vi "beginDirectKickPlay.vi"(8 "error in (no error)":errorcluster, 10 "Game":refnum<class "Game.lvclass">, 11 "DirectKickPlay in":refnum<class "DirectKickPlay.lvclass">) -> (0 "error out":errorcluster, 2 "directKickBegin?":bool, 3 "DirectKickPlay out":refnum<class "DirectKickPlay.lvclass">)   [LabVIEW 2018, in "DirectKickPlay.lvclass"]
uses:
  DirectKickPlay.lvclass
  Game_class/Game.lvclass
  Utilities_class/Utilities.lvclass
  Referee_class/command_interpreted.ctl
  Team_class/OffensivePlay.ctl
  Game_class/Game.lvclass/Game.ctl
  Referee_class/Referee.lvclass/Referee.ctl
  Team_class/Team.lvclass/Team.ctl
  Game_class/Read OffensiveTeam.vi
  Team_class/Read OffensivePlay.vi
  Game_class/Read Referee.vi
  Referee_class/Read command_interpreted.vi
  Ally_class/Ally.lvclass
  Referee_class/Referee.lvclass
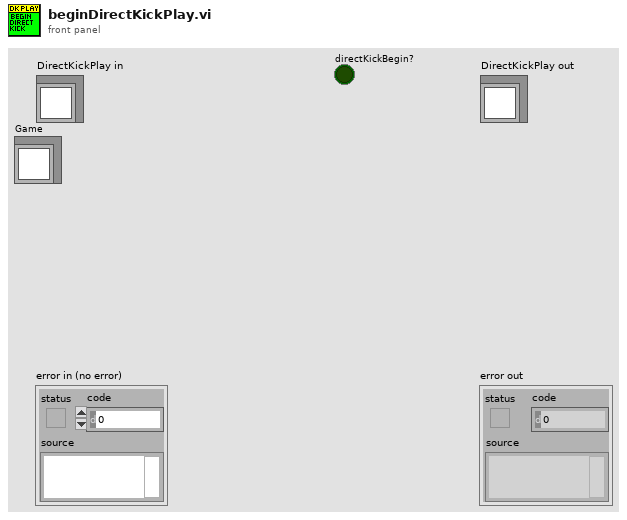
[diagram p1: front panel]
types:
  T1 = typedef "OffensivePlay.ctl" = enum16{"PreparePass", "PassToStriker", "BallOutOfField", "PassTo2ndStriker", "StopOffensive", "Prepare Penalty Enemy", "EnemyPossessionAtEnemyField", "EnemyPossesionAtOurField", "TestPlay", "PreparePenaltyAlly", "KickPenaltyAlly", "PrepareKickoffAlly", "PrepareKickoffEnemy", "IndirectEnemy", "DirectEnemy", "NormalGame", "DirectKick", "Pass", "Halt", "Timeout", "PassPlay", "PenaltyEnemy", "SimplePass"}
  T2 = typedef "command_interpreted.ctl" = enum16{"Goal Ally", "Goal Enemy", "Ball Placement Enemy", "Ball Placement Ally", "Normal Half Time", "Extra Time  Break", "Extra Half Time", "None", "Post Game", "PKA Normal Start", "Prepare Kickoff Ally", "PKE Normal Start", "Prepare Kickoff Enemy", "Force Start", "Halt", "Timeout", "Prepare Penalty Ally", "Prepare Penalty Enemy", "PPA NormalStart", "PPE Normal Start", "Indirect Free Ally", "Direct Free Enemy", "Direct Free Ally", "Indirect Free Enemy", "Stop"}
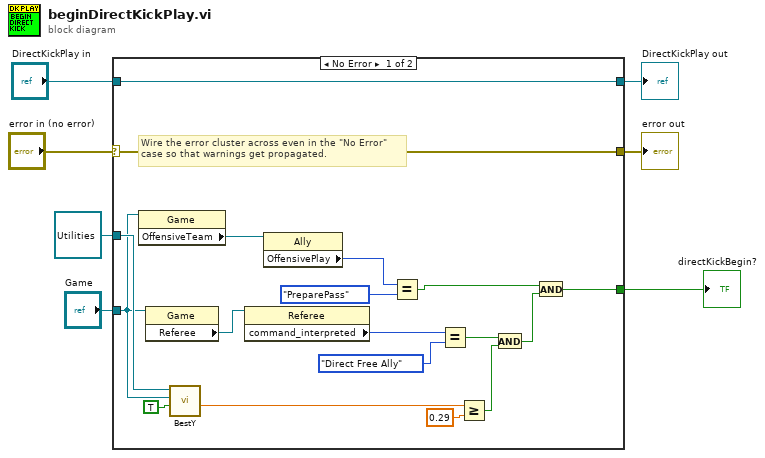
[diagram p0: block diagram]
diagram:
  n1 = case shown="No Error" "error in (no error)" {
    selector: "error in (no error)" -> [w24 w27]
    tunnel: [w24 w27] -> w6
    tunnel: [w25 w26] -> w4
    tunnel: "DirectKickPlay in" -> [w25 w26]
    tunnel: "Game" -> [w12 _]
    tunnel: refnum<class "Utilities.lvclass"> refnum ("Utilities.lvclass") -> [w19 _]
    tunnel: [w10 _] -> w1
    frame No Error {
      # "Wire the error cluster across even in the \"No Error\"\ncase so that warnings get propagated."
      n2 = property class="Game"(reference=w12) -> ("OffensiveTeam"=w14:refnum<class "Ally.lvclass">)  [unwired: 1 in, 2 out]
      n3 = property class="Game"(reference=w12) -> ("Referee"=w23:refnum<class "Referee.lvclass">)  [unwired: 1 in, 2 out]
      n4 = call-dynamic "BestY.vi"("Utilities in"=w19, "Game"=w12, "inimigos"=TRUE) -> ("Gap kick"=w18:dbl)  [unwired: 2 in, 4 out]
      n5 = property class="Referee"(reference=w23) -> ("command_interpreted"=w22:T2)  [unwired: 1 in, 2 out]
      n6 = property class="Ally"(reference=w14) -> ("OffensivePlay"=w9:T1)  [unwired: 1 in, 2 out]
      n7 = Equal?(x=w9, y=OffensivePlay."PreparePass" ("OffensivePlay")) -> (x = y?=w8:bool)
      n8 = Equal?(x=w22, y=command_interpreted."Direct Free Ally" ("command_interpreted")) -> (x = y?=w16:bool)
      n9 = Greater Or Equal?(x=w18, y=0.29 ("Gap kick")) -> (x >= y?=w15:bool)
      n10 = And(x=w16, y=w15) -> (x .and. y?=w11:bool)
      n11 = And(x=w8, y=w11) -> (x .and. y?=w10:bool)
    }
    frame Error {
    }
  }
  "error out" <- w6
  "DirectKickPlay out" <- w4
  "directKickBegin?" <- w1
